vi "LowTransport.vi"(5 "LogSuspend":bool, 8 "error in":errorcluster, 10 "Request":u8[](array[numeric]) format="%02x", 11 "HandleIn":T1={"LogPath"=path "", "LogEnabled"=FALSE, "isOpen"=FALSE, "LogContent"="", "Adapter"="CAN0", "MCanHandle"={"MCanAdapter"=refnum}, "TransmittId"=0, "ReceiveId"=0}) -> (0 "error out":errorcluster, 2 "Response":u8[](array[numeric]) format="%02x", 3 "HandleOut":T1={"LogPath"=path "", "LogEnabled"=FALSE, "isOpen"=FALSE, "LogContent"="", "Adapter"="CAN0", "MCanHandle"={"MCanAdapter"=refnum}, "TransmittId"=0, "ReceiveId"=0})   [LabVIEW 2011, in "Konvolucio MUDS150628.lvlib"]
uses:
  <instrlib>/Konvolucio MUDS150628/Konvolucio MUDS150628.lvlib
  <instrlib>/Konvolucio MUDS150628/Types/UdsHandleType.ctl
  <instrlib>/Konvolucio MCAN120803/Types/MCanHandleType.ctl
  C:/Program Files/National Instruments/LabVIEW 2011/instr.lib/Konvolucio MCAN120803/Private/Konvolucio.MCAN120803.dll
  Konvolucio MCAN120803/Private/Konvolucio.MCAN120803.dll
  <instrlib>/Konvolucio MUDS150628/Private/UdsLogEvent.vi
  <instrlib>/Konvolucio MUDS150628/Private/UdsLogErrorCheckPoint.vi
  <instrlib>/Konvolucio MCAN120803/Konvolucio MCAN120803.lvlib
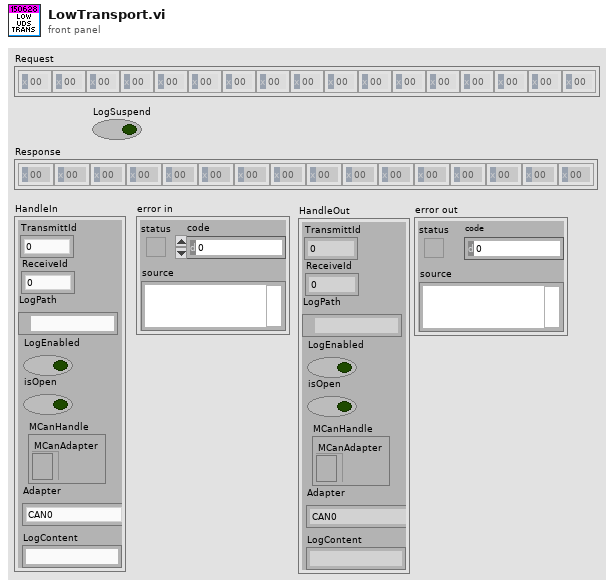
[diagram p1: front panel]
types:
  T1 = typedef "Konvolucio MUDS150628.lvlib/UdsHandleType.ctl" = cluster{"LogPath":path, "LogEnabled":bool, "isOpen":bool, "LogContent":string, "Adapter":string, "MCanHandle":T2, "TransmittId":u32, "ReceiveId":u32}
  T2 = typedef "Konvolucio MCAN120803.lvlib/MCanHandleType.ctl" = cluster{"MCanAdapter":refnum<k24>}
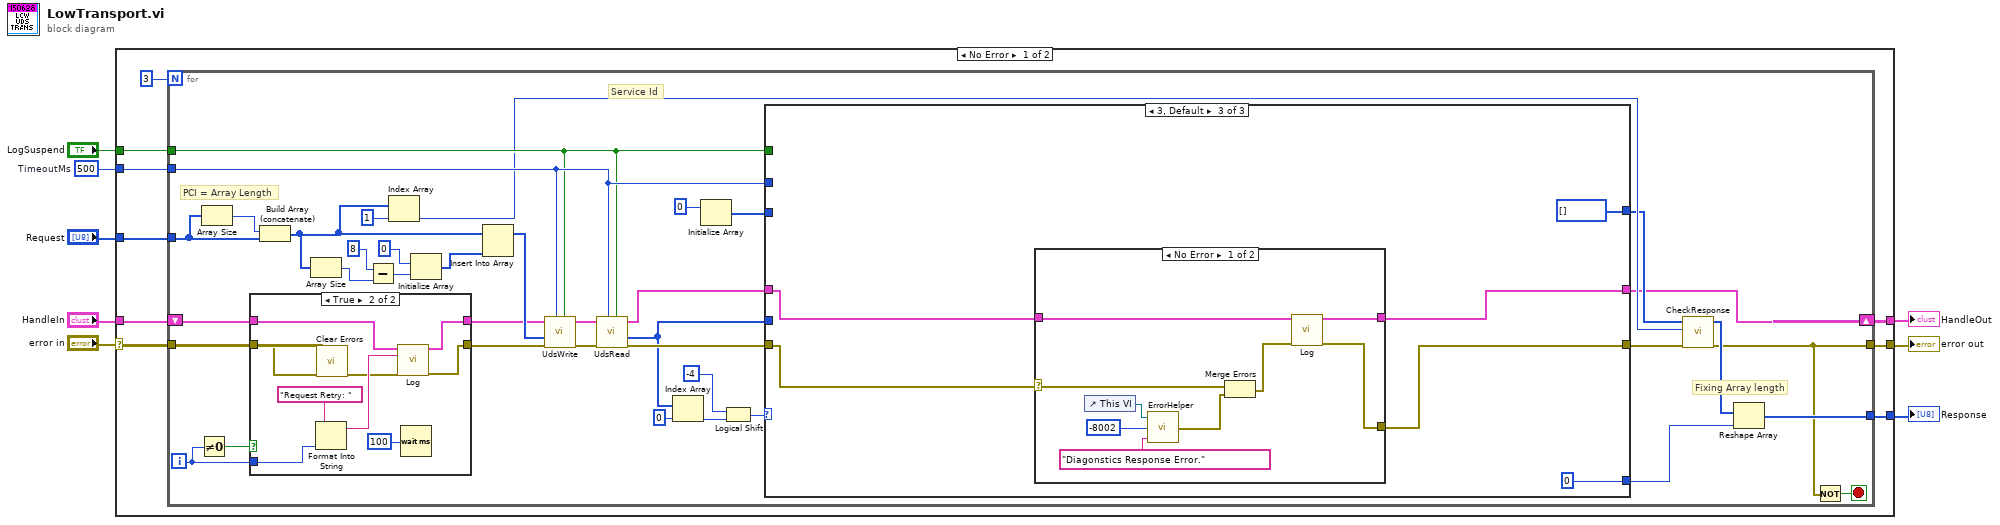
[diagram p0: block diagram]
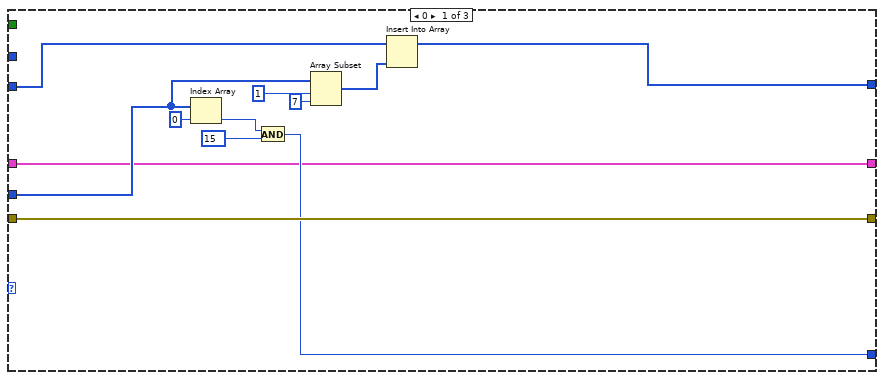
[diagram p3: hidden frame]
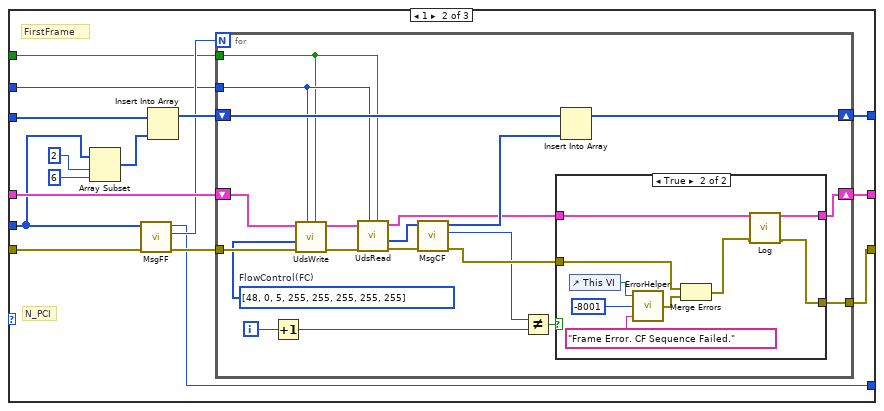
[diagram p4: hidden frame]
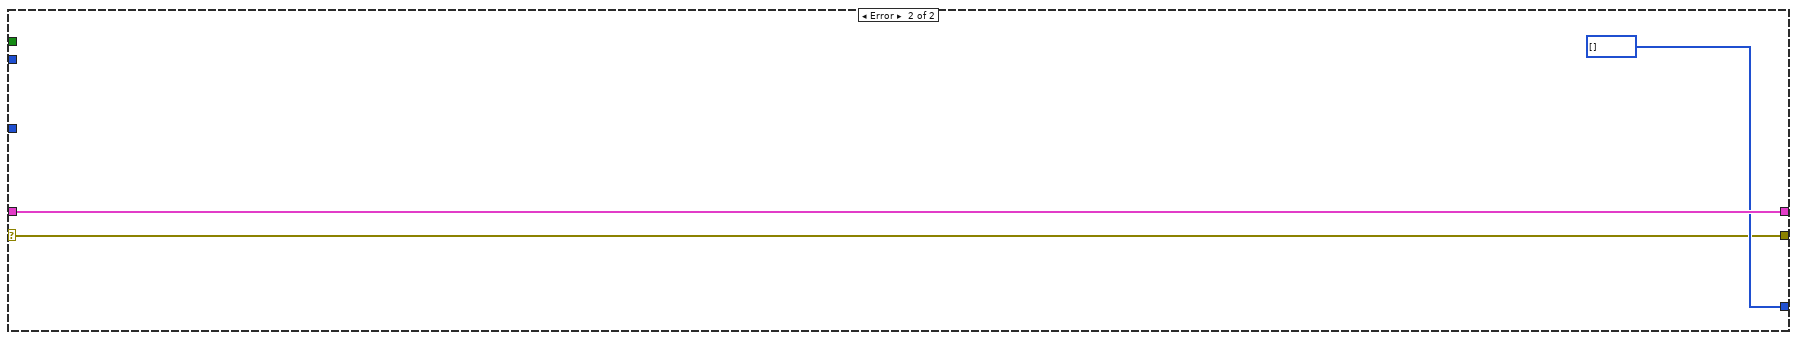
[diagram p7: hidden frame]
diagram:
  w4 = u32 500  # TimeoutMs
  n1 = case shown="No Error" "error in" {
    selector: "error in" -> [w13 w143]
    tunnel: "HandleIn" -> [w16 w145]
    tunnel: [w17 w143] -> w7
    tunnel: [w9 w145] -> w6
    tunnel: [w11 u8[] []] -> w2
    tunnel: "Request" -> [w12 _]
    tunnel: w4 -> [w15 _]
    tunnel: "LogSuspend" -> [w14 _]
    frame No Error {
      n2 = for {
        N: 3 -> [_]
        tunnel: [w18] -> w17
        tunnel: w15 -> [w45]
        tunnel: w14 -> [w44]
        tunnel: w13 -> [w21]
        tunnel: w12 -> [w40]
        tunnel: [w29] -> w11
        shift-right: [w19] -> w9
        shift-left: w16 -> [w24]
        i -> [w23]
        stop <- w26 stop-if-true
        # "Fixing Array length"
        # "PCI = Array Length"
        # "Service Id"
        n3 = Not Equal To 0?(x=w23) -> (x != 0?=w25:bool)
        n4 = Array Size(array=w40) -> (size(s)=w39:i32)
        n5 = case shown="True" w25 {
          tunnel: w24 -> [w57 w59]
          tunnel: w23 -> [_ w65]
          tunnel: [w57 w58] -> w22
          tunnel: w21 -> [w56 w64]
          tunnel: [w56 w60] -> w20
          frame False {
          }
          frame True {
            n6 = Format Into String(initial string="Request Retry: ", w65) -> (resulting string=w62:string)  [unwired: 2 in, 1 out]
            n7 = call <vilib>:"Clear Errors.vi"("error in (no error)"=w64) -> ("error out"=w61:errorcluster)  [unwired: 6 in]
            n8 = call-poly <instrlib>:"Log.vi"("UdsHandleIn"=w59, "EventMsg"=w62, "error in"=w61) -> ("UdsHandleOut"=w58:T1, "error out"=w60:errorcluster)  [unwired: 11 in]
            n9 = Wait (ms)(milliseconds to wait=u32 100) -> ()  [unwired: 1 out]
          }
        }
        n10 = Build Array (concatenate)(w39, w40) -> (w34:i32[])
        n11 = Array Size(array=w34) -> (size(s)=w38:i32)
        n12 = Subtract(x=8, y=w38) -> (x-y=w36:i32)
        n13 = Index Array(array=w34, index=1) -> (element=w42:i32)
        n14 = Initialize Array(u8 0 ("index"), w36) -> (w33:u8[])
        n15 = Insert Into Array(array=w34, new element=w33) -> (w32:i32[])  [unwired: 1 in]
        n16 = call <instrlib>:"UdsWrite.vi"("LogSuspend"=w44, "TimeoutMs"=w45, "error in"=w20, "DataIn"=w32, "UdsHandleIn"=w22) -> ("error out"=w49:errorcluster, "UdsHandleOut"=w48:T1)  [unwired: 5 in]
        n17 = call <instrlib>:"UdsRead.vi"("LogSuspend"=w44, "TimeoutMs"=w45, "error in"=w49, "UdsHandleIn"=w48) -> ("error out"=w47:errorcluster, "Data"=w27:u8[], "UdsHandleOut"=w46:T1)  [unwired: 5 in]
        n18 = Index Array(array=w27, index=0) -> (element=w53:u8)
        n19 = Initialize Array(u8 0 ("dimension size")) -> (w50:u8[])  [unwired: 1 in]
        n20 = Logical Shift(y=-4 ("x"), x=w53) -> (x << y=w52:u8)
        n21 = case shown="3, Default" w52 {
          tunnel: w27 -> [w68 w83 _]
          tunnel: w47 -> [w78 w94 w128]
          tunnel: w46 -> [w67 w92 w127]
          tunnel: w45 -> [_ w81 _]
          tunnel: [w78 w79 w129] -> w41
          tunnel: [w74 w85 0 ("FF_DL")] -> w30
          tunnel: [w69 w88 u8[] []] -> w28
          tunnel: w50 -> [w70 w84 _]
          tunnel: [w67 w82 w126] -> w19
          tunnel: w44 -> [_ w80 _]
          frame 0 {
            n22 = Index Array(array=w68, index=0) -> (element=w76:u8)
            n23 = And(x=w76, y=15) -> (x .and. y?=w74:i32)
            n24 = Array Subset(array=w68, index=1, length=7) -> (w71:u8[])
            n25 = Insert Into Array(array=w70, new element=w71) -> (w69:u8[])  [unwired: 1 in]
          }
          frame 1 {
            # "N_PCI"
            # "FirstFrame"
            n26 = Array Subset(array=w83, index=2, length=6) -> (w89:u8[])
            n27 = call <instrlib>:"MsgFF.vi"("error in"=w94, "Data"=w83) -> ("error out"=w93:errorcluster, "CF_Count"=w86:i32, "FF_DL"=w85:i32)  [unwired: 7 in]
            n28 = Insert Into Array(array=w84, new element=w89) -> (w87:u8[])  [unwired: 1 in]
            n29 = for {
              N: w86 -> [_]
              tunnel: w93 -> [w107]
              tunnel: [w111] -> w79
              shift-right: [w109] -> w88
              shift-left: w87 -> [w110]
              tunnel: w81 -> [w101]
              tunnel: w80 -> [w100]
              shift-right: [w95] -> w82
              shift-left: w92 -> [w106]
              i -> [w114]
              w105 = u8[] [48, 0, 5, 255, 255, 255, 255, 255]  # FlowControl(FC)
              n30 = Increment(x=w114) -> (x+1=w98:i32)
              n31 = call <instrlib>:"UdsWrite.vi"("LogSuspend"=w100, "TimeoutMs"=w101, "error in"=w107, "DataIn"=w105, "UdsHandleIn"=w106) -> ("error out"=w104:errorcluster, "UdsHandleOut"=w103:T1)  [unwired: 5 in]
              n32 = call <instrlib>:"UdsRead.vi"("LogSuspend"=w100, "TimeoutMs"=w101, "error in"=w104, "UdsHandleIn"=w103) -> ("error out"=w102:errorcluster, "Data"=w99:u8[], "UdsHandleOut"=w96:T1)  [unwired: 5 in]
              n33 = call <instrlib>:"MsgCF.vi"("error in"=w102, "DataIn"=w99) -> ("error out"=w112:errorcluster, "SN"=w97:i32, "CF Data Bytes"=w108:u8[])  [unwired: 7 in]
              n34 = Not Equal?(x=w97, y=w98) -> (x != y?=w113:bool)
              n35 = case shown="True" w113 {
                tunnel: w112 -> [w116 w125]
                tunnel: [w116 w117] -> w111
                tunnel: w96 -> [w115 w120]
                tunnel: [w115 w119] -> w95
                frame False {
                }
                frame True {
                  n36 = control-ref of="This VI"() -> (w124:refnum<vi>)
                  n37 = call <instrlib>:"ErrorHelper.vi"("Message"="Frame Error. CF Sequence Failed.", "Code"=-8001 ("code"), "This VI"=w124) -> ("error out"=w122:errorcluster)
                  n38 = Merge Errors(w125, w122) -> (w118:errorcluster)
                  n39 = call-poly <instrlib>:"Log.vi"("UdsHandleIn"=w120, "error in"=w118) -> ("UdsHandleOut"=w119:T1, "error out"=w117:errorcluster)  [unwired: 12 in]
                }
              }
              n40 = Insert Into Array(array=w110, new element=w108) -> (w109:u8[])  [unwired: 1 in]
            }
          }
          frame 3, Default {
            n41 = case shown="No Error" w128 {
              selector: w128 -> [w140 w142]
              tunnel: [w132 w142] -> w129
              tunnel: w127 -> [w134 w141]
              tunnel: [w135 w141] -> w126
              frame No Error {
                n42 = control-ref of="This VI"() -> (w137:refnum<vi>)
                n43 = call <instrlib>:"ErrorHelper.vi"("Message"="Diagonstics Response Error.", "Code"=-8002 ("code"), "This VI"=w137) -> ("error out"=w136:errorcluster)
                n44 = Merge Errors(w140, w136) -> (w133:errorcluster)
                n45 = call-poly <instrlib>:"Log.vi"("UdsHandleIn"=w134, "error in"=w133) -> ("UdsHandleOut"=w135:T1, "error out"=w132:errorcluster)  [unwired: 12 in]
              }
              frame Error {
              }
            }
          }
        }
        n46 = call <instrlib>:"CheckResponse.vi"("error in"=w41, "SID"=w42, "DataIn"=w28) -> ("error out"=w18:errorcluster, "DataOut"=w31:u8[])  [unwired: 7 in]
        n47 = Reshape Array(w31, w30) -> (w29:u8[])
        n48 = Not(x=w18) -> (.not. x?=w26:bool)
      }
    }
    frame Error {
    }
  }
  "HandleOut" <- w6
  "error out" <- w7
  "Response" <- w2
